vi "Map Graph Coords.vi"(8 "error in (no error)":errorcluster, 9 "XY":cluster{dbl, dbl}, 11 "Timeline Graph in":refnum<vi>) -> (0 "error out":errorcluster, 1 "Coords":cluster{i32, i32})   [LabVIEW 2020, in "XGrapher.xctl"]
uses:
  XGrapher.xctl
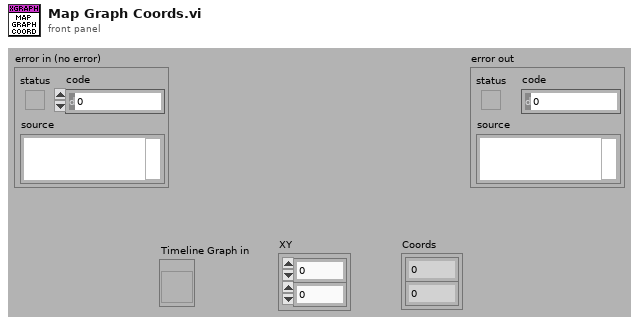
[diagram p1: front panel]
types:
  T1 = typedef "LVRectTypeDef.ctl" = cluster{"Left":i16, "Top":i16, "Right":i16, "Bottom":i16}
  T2 = typedef "LVPoint32TypeDef.ctl" = cluster{"Horizontal":i32, "Vertical":i32}
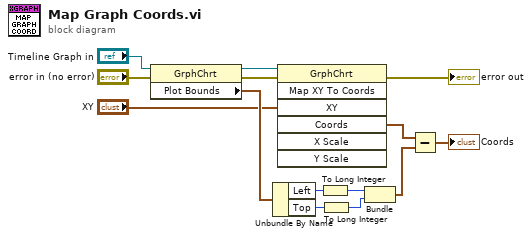
[diagram p0: block diagram]
diagram:
  n1 = property on="Property Node" class="GrphChrt"(reference="Timeline Graph in", error in="error in (no error)") -> (reference out=w6:refnum<vi>, error out=w9:errorcluster, "Plot Bounds"=w12:T1)
  n2 = Unbundle By Name(w12) -> ("Left"=w13:i16, "Top"=w14:i16)
  n3 = invoke on="Invoke Node" class="GrphChrt" method="Map XY To Coords"(reference=w6, error in=w9, "XY"="XY") -> (error out=→"error out":errorcluster, "Coords"=w5:T2)  [unwired: 4 in, 5 out]
  n4 = To Long Integer(number=w13) -> (32bit integer=w4:i32)
  n5 = To Long Integer(number=w14) -> (32bit integer=w3:i32)
  n6 = Bundle(w4, w3) -> (w2:cluster{i32, i32})  [unwired: 1 in]
  n7 = Subtract(x=w5, y=w2) -> (x-y=→"Coords":T2)
